vi "AddControlPressure2Psequence.vi"(9 "Control Pressure":dbl=300.0, 10 "Ctr Pressure Channel":u16=1, 11 "Psequence":dbl[][](array[numeric])=[[nan, 901.0, 850.0, 840.0], [nan, 950.0, 850.0, 840.0]]) -> (3 "Psequence Out":dbl[][](array[numeric]))   [LabVIEW 2016]
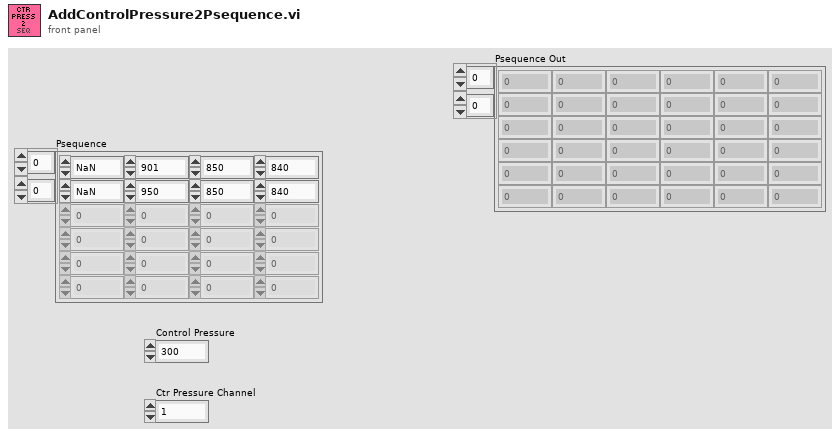
[diagram p1: front panel]
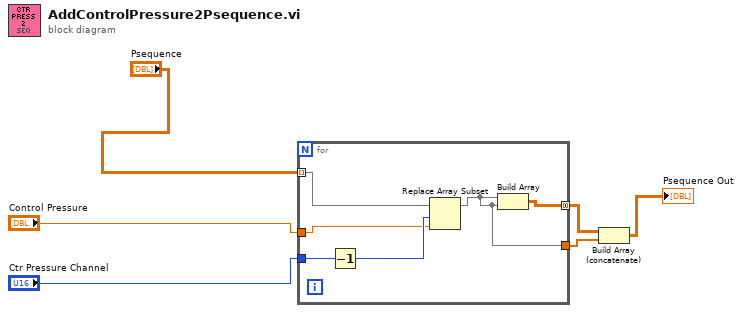
[diagram p0: block diagram]
diagram:
  n1 = for {
    tunnel: "Psequence" -> [w12] mode=indexing
    tunnel: "Ctr Pressure Channel" -> [w11]
    tunnel: "Control Pressure" -> [w9]
    tunnel: [w8] -> w3 mode=concatenating
    tunnel: [w7] -> w2
    n2 = Decrement(x=w11) -> (x-1=w10:u16)
    n3 = Replace Array Subset(array=w12, new element=w9, index=w10) -> (w7:dbl[])
    n4 = Build Array(w7, w7) -> (w8:dbl[][])
  }
  n5 = Build Array (concatenate)(w3, w2) -> (→"Psequence Out":dbl[][])
